vi "MGCC_FntStaMach_FlagCalculate_PhaseTwo.vi"(10 "Current SubMG":i32[](array[numeric]), 11 "Input State":string[](array[string])) -> (3 "Output Event":bool[][](array[boolean]))   [LabVIEW 2016]
uses:
  MGCC_FntStaMach_gobal.vi
  <vilib>/imath/engines/lvmath2/RunTimeEngine/IndexRead/NIMS M(S,$).vi
  <instcachedir>/0/NIMS M(S,$)_F24F360562DE41D8BE234322A2E15C65.lvgen/NIMS M(S,$)_F24F360562DE41D8BE234322A2E15C65_000.vi
  <vilib>/imath/engines/lvmath2/RunTimeEngine/BuiltInFunctions/length/NIMS_length(GV).vi
  <instcachedir>/0/NIMS_length(GV)_08A3D13377FD4E4B96F5795FBF3698FA.lvgen/NIMS_length(GV)_08A3D13377FD4E4B96F5795FBF3698FA_000.vi
  <vilib>/imathl/engines/lvmath/Functions/Error Handling/Create Error.vi
  <vilib>/imath/engines/lvmath2/RunTimeEngine/RangeToken/NIMS_Range_R3 - Integer.vi
  <instcachedir>/0/NIMS_Range_R3 - Integer_A435E2FF893B4C718FD5055FE39FE2F6.lvgen/NIMS_Range_R3 - Integer_A435E2FF893B4C718FD5055FE39FE2F6_000.vi
  <vilib>/imath/engines/lvmath2/RunTimeEngine/CommandStatement/MC_CommandStatement_break.vi
  <vilib>/imath/engines/lvmath2/RunTimeEngine/IndexRead/NIMS M(S,S).vi
  <instcachedir>/0/NIMS M(S,S)_AC51E74150A542F7991B9634C66F3096.lvgen/NIMS M(S,S)_AC51E74150A542F7991B9634C66F3096_000.vi
  <vilib>/imath/engines/lvmath2/RunTimeEngine/BuiltInFunctions/findnz/NIMS_[1o]_findnz(GRowV).vi
  <instcachedir>/0/NIMS_[1o]_findnz(GRowV)_1AF74843B4874134ADE908C0A4A72F3C.lvgen/NIMS_[1o]_findnz(GRowV)_1AF74843B4874134ADE908C0A4A72F3C_000.vi
  <vilib>/imath/engines/lvmath2/RunTimeEngine/BuiltInFunctions/is_empty/NIMS_is_empty(GV).vi
  <instcachedir>/0/NIMS_is_empty(GV)_FC7E7C3D9544432CB6AA2416ADCF6D56.lvgen/NIMS_is_empty(GV)_FC7E7C3D9544432CB6AA2416ADCF6D56_000.vi
  <vilib>/imath/engines/lvmath2/RunTimeEngine/ErrorHandling/NIMS_Create Error From Enums.vi
  <vilib>/imath/engines/lvmath2/RunTimeEngine/NodeEndStatement/NIMS_NodeEndStatement_Output.vi
  <instcachedir>/0/NIMS_NodeEndStatement_Output_53EC0D466D134D7ABD903AC30B43404B.lvgen/NIMS_NodeEndStatement_Output_53EC0D466D134D7ABD903AC30B43404B_013.vi
  <vilib>/imath/engines/lvmath2/RunTimeEngine/ErrorHandling/NIMS_Finalize Error.vi
panel:
  in  "ISD":bool
  out "Current SubMG":dbl
  out "Error Array":errorcluster[](array[cluster])
  in  "Ready for the next MG":bool
  in  "FLT 10":bool
  in  "ABN 10":bool
  in  "STD 6":bool
  in  "FLT 9":bool
  in  "ABN 9":bool
  in  "STD 5":bool
  in  "OFF":bool
  in  "GC 4":bool
  in  "ISD 6":bool
  in  "G2I_UN 3":bool
  in  "G2I_IN 3":bool
  in  "STD 4":bool
  in  "I2G 3":bool
  in  "BKS 3":bool
  in  "ABN 8":bool
  in  "FLT 8":bool
  in  "STD 3":bool
  in  "BKS 2":bool
  in  "ABN 7":bool
  in  "FLT 7":bool
  in  "ISD 5":bool
  in  "STD  3":bool
  in  "I2G 2":bool
  in  "ABN 6":bool
  in  "FLT 6":bool
  in  "GC 3":bool
  in  "STD 2":bool
  in  "ISD 4":bool
  in  "ABN 5":bool
  in  "FLT 5":bool
  in  "G2I_UN 2":bool
  in  "STD  2":bool
  in  "ISD 3":bool
  in  "ABN 4":bool
  in  "FLT 4":bool
  in  "G2I_IN 2":bool
  in  "I2G":bool
  in  "ISD 2":bool
  in  "ABN 3":bool
  in  "FLT 3":bool
  in  "GC 2":bool
  in  "G2I_UN":bool
  in  "G2I_IN":bool
  in  "ABN 2":bool
  in  "FLT 2":bool
  in  "GC":bool
  in  "ISD":bool
  in  "BKS":bool
  in  "STD":bool
  in  "ABN":bool
  in  "FLT":bool
  # "OFF State"
  # "STD State"
  # "GC State"
  # "BKS State"
  # "ISD State"
  # "ABN State"
  # "G2I_UN State"
  # "G2I_IN State"
  # "FLT State"
  # "I2G State"
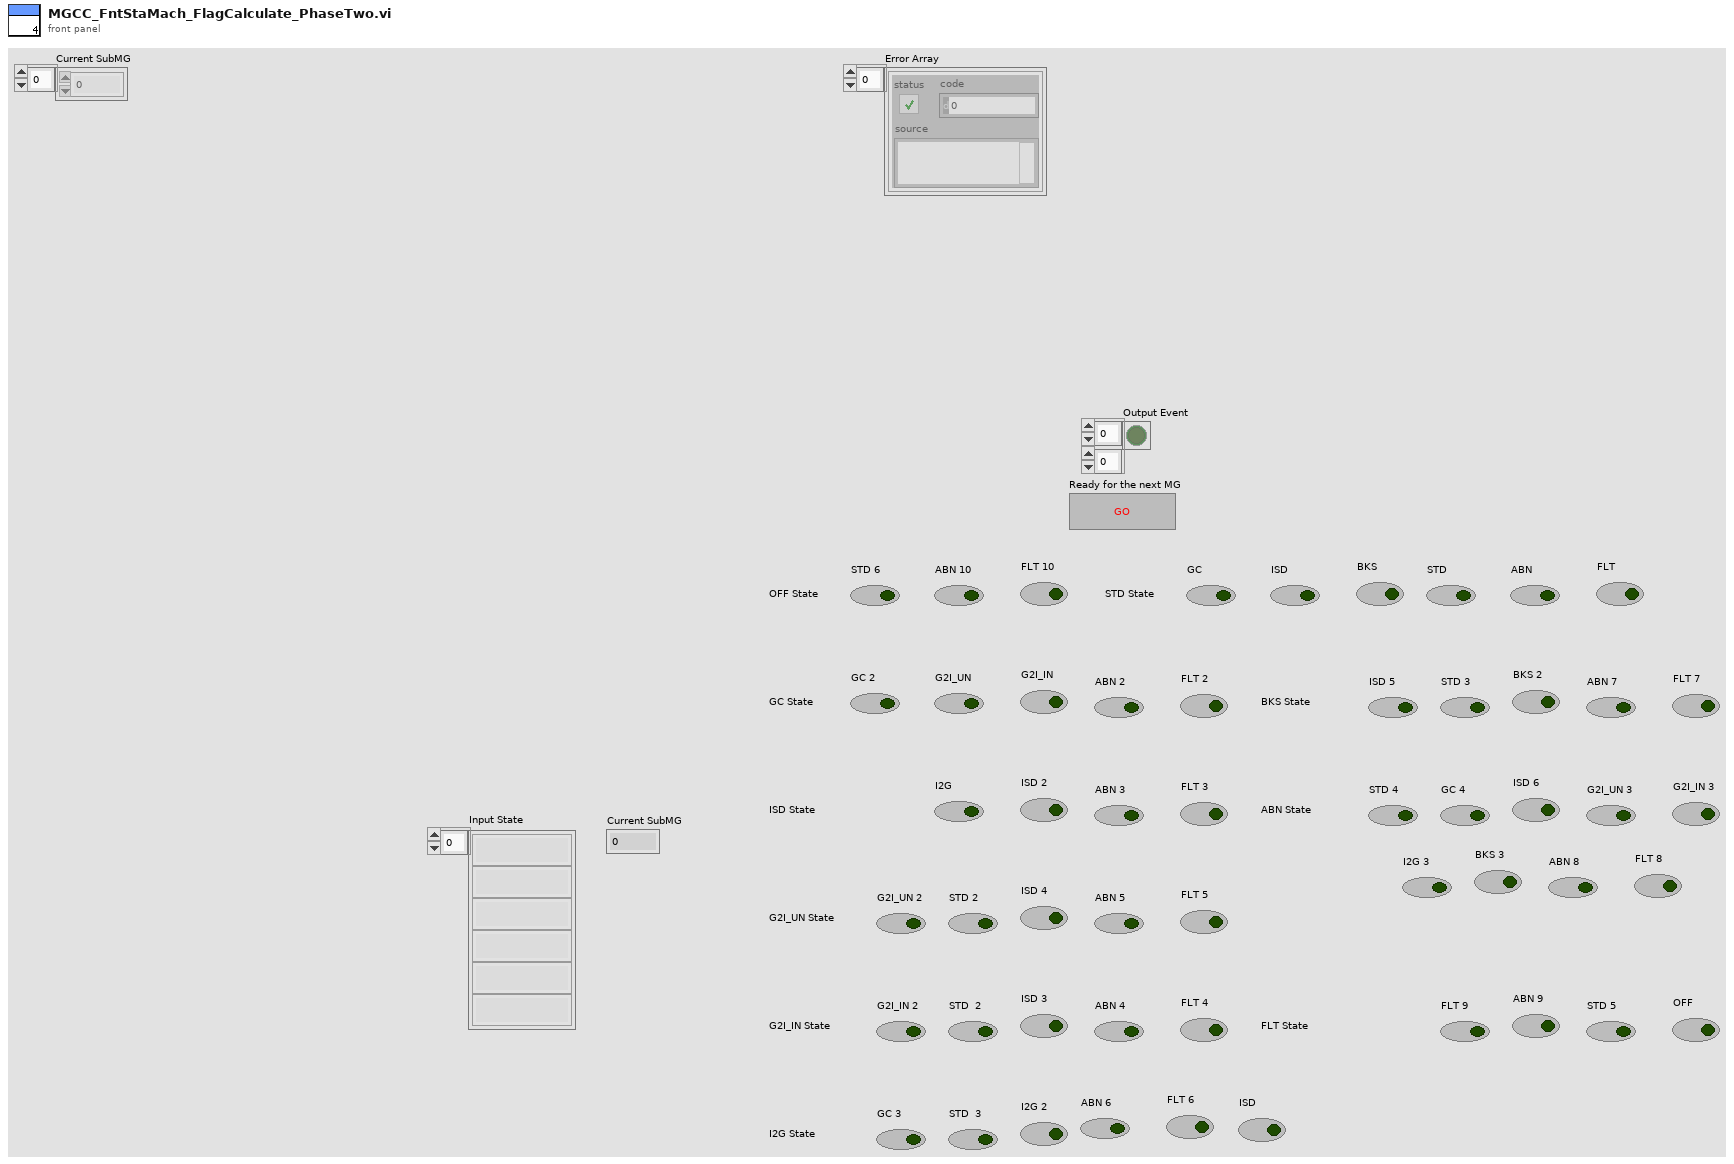
[diagram p1: front panel]
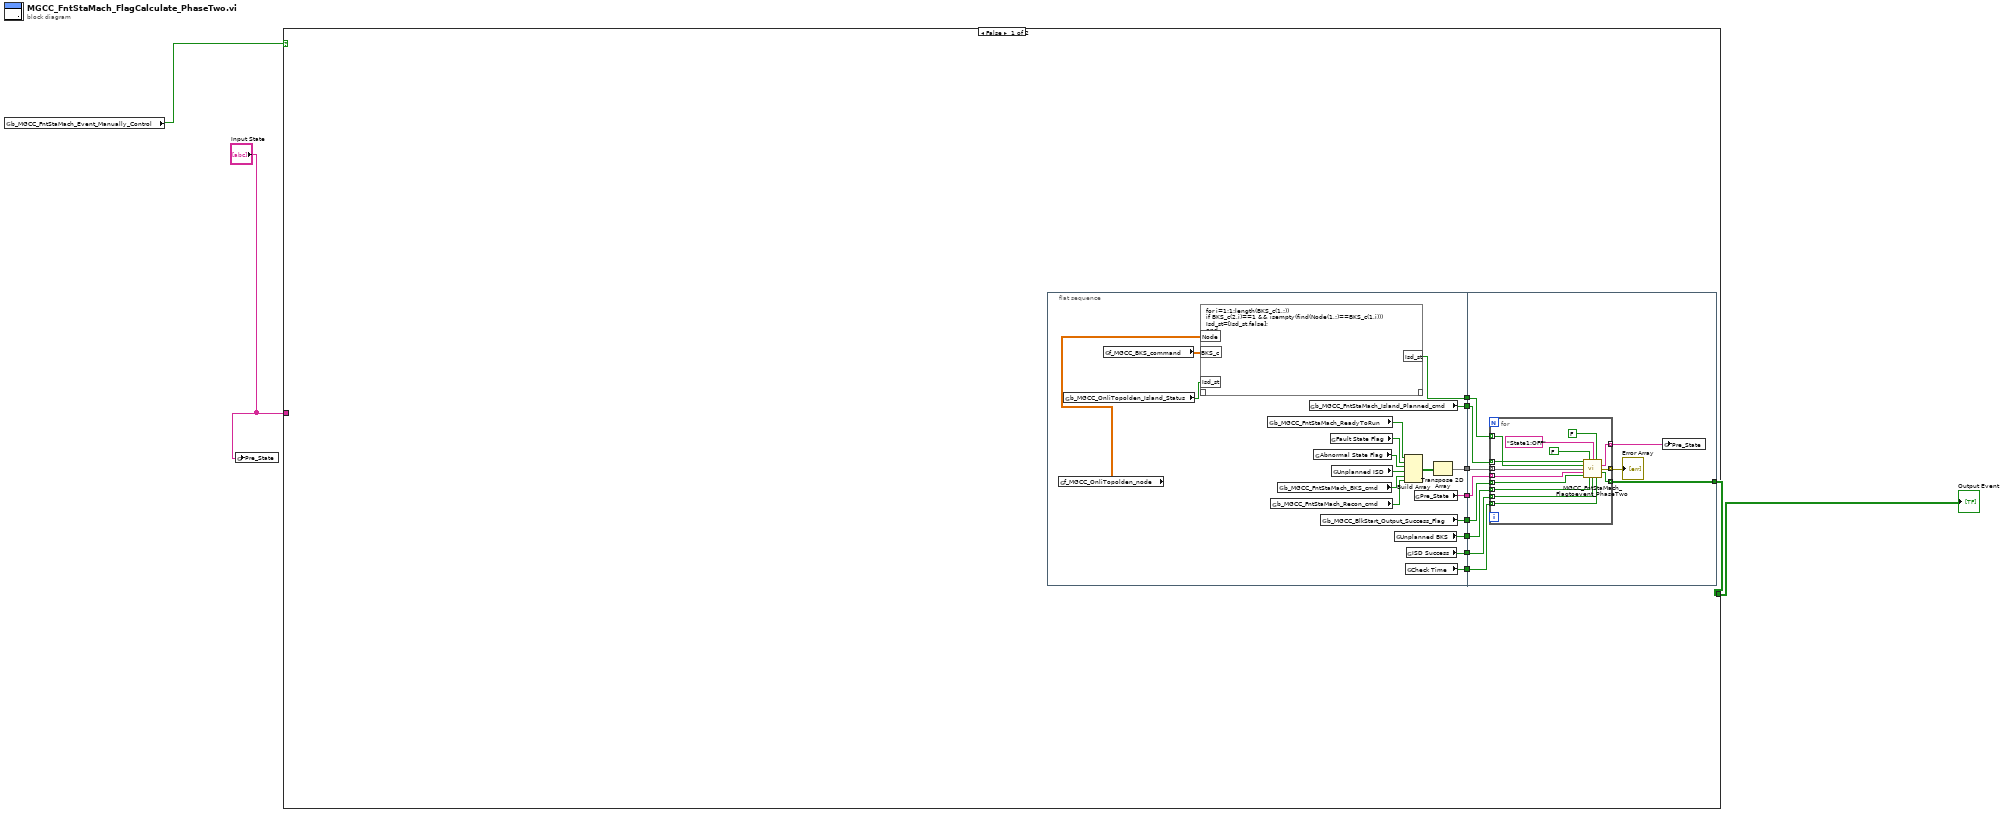
[diagram p0: block diagram]
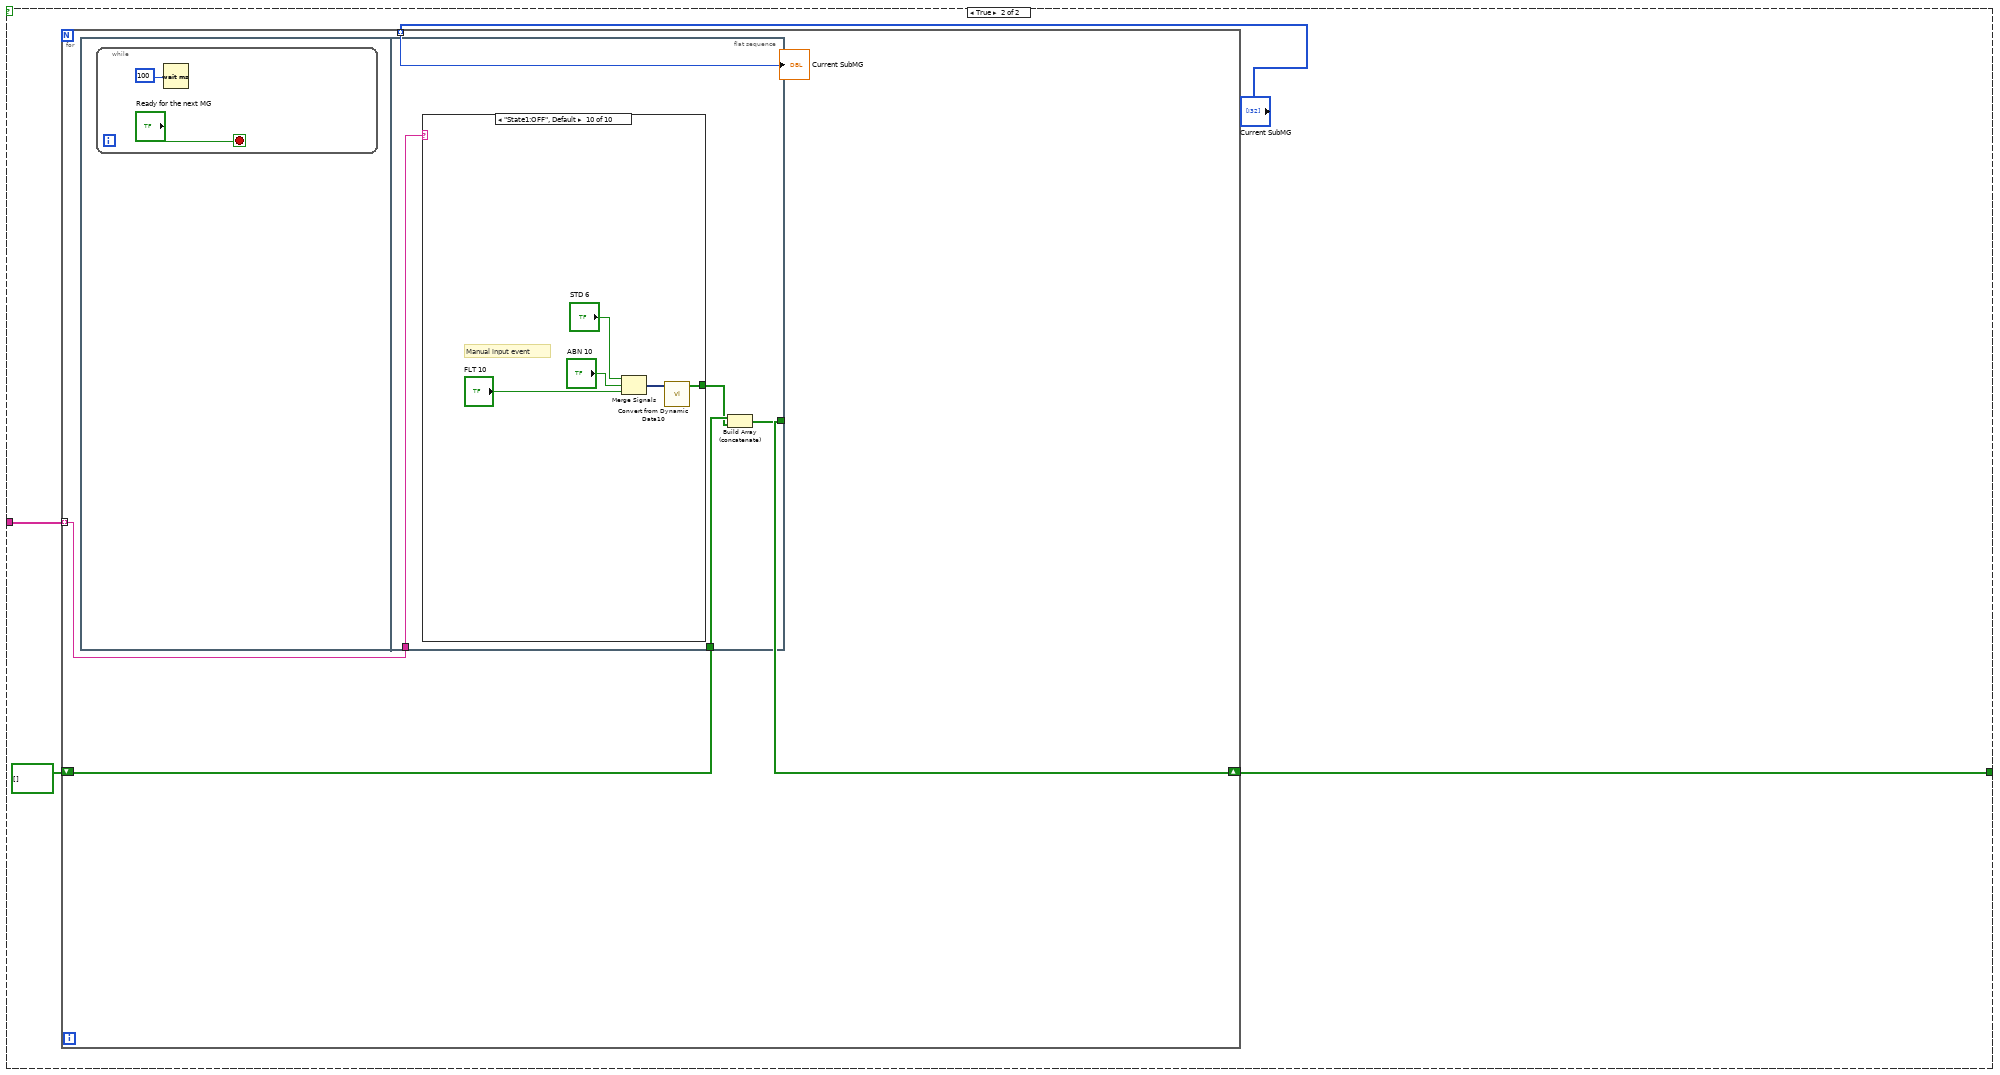
[diagram p2: hidden frame]
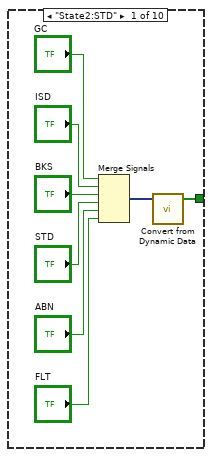
[diagram p3: hidden frame]
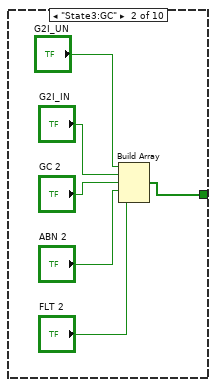
[diagram p4: hidden frame]
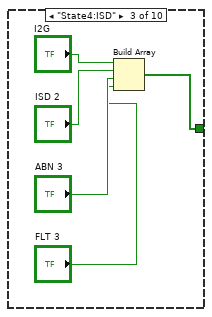
[diagram p5: hidden frame]
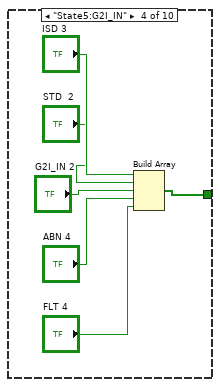
[diagram p6: hidden frame]
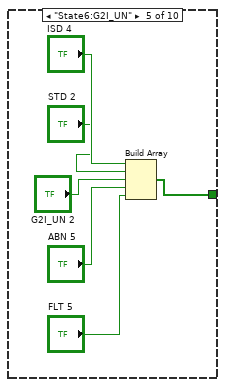
[diagram p7: hidden frame]
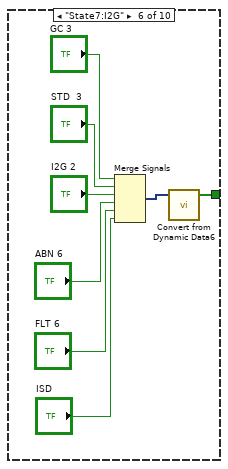
[diagram p8: hidden frame]
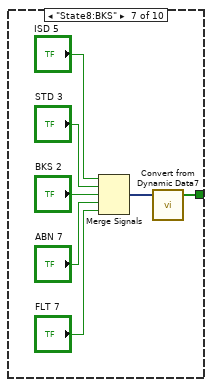
[diagram p9: hidden frame]
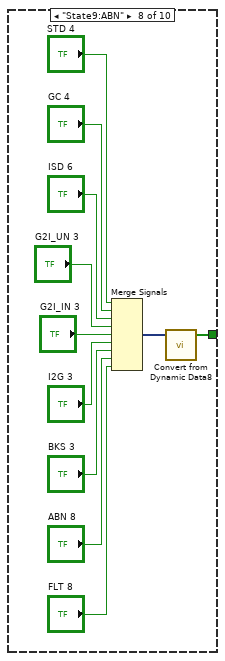
[diagram p10: hidden frame]
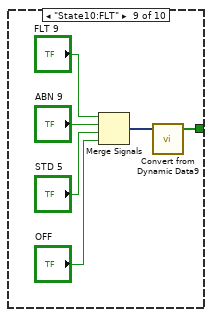
[diagram p11: hidden frame]
diagram:
  n1 = global read "MGCC_FntStaMach_gobal.vi" "b_MGCC_FntStaMach_Event_Manually_Control"() -> (w3:bool)
  n2 = global write "MGCC_FntStaMach_gobal.vi" "Pre_State"("Input State") -> ()
  n3 = case shown="False" w3 {
    tunnel: "Input State" -> [_ w197]
    tunnel: [w4 w194] -> w2
    frame False {
      n4 = flat-sequence {
        tunnel: [w17] -> w12
        tunnel: [w24] -> w11
        tunnel: [w14] -> w10
        tunnel: [w23] -> w9
        tunnel: [w22] -> w8
        tunnel: [w21] -> w7
        tunnel: [w20] -> w6
        tunnel: [w19] -> w5
        tunnel: w12 -> [w179]
        tunnel: w11 -> [w178]
        tunnel: w10 -> [w177]
        tunnel: w9 -> [w176]
        tunnel: w8 -> [w175]
        tunnel: w7 -> [w174]
        tunnel: w6 -> [w173]
        tunnel: w5 -> [w172]
        tunnel: [w170] -> w4
        frame #0 {
          n5 = global read "MGCC_FntStaMach_gobal.vi" "f_MGCC_OnliTopolden_node"() -> (w13:dbl[][])
          n6 = global read "MGCC_FntStaMach_gobal.vi" "b_MGCC_OnliTopolden_Island_Status"() -> (w15:bool[])
          n7 = global read "MGCC_FntStaMach_gobal.vi" "f_MGCC_BKS_command"() -> (w16:dbl[][])
          n8 = mathscript code="for i=1:1:length(BKS_c(1,:))\nif BKS_c(2,i)==1 && isempty(find(Node(1,:)==BKS_c(1,i)))\nIsd_st=[Isd_st,false];\nend\nend"("BKS_c"=w16, "Isd_st"=w15, "Node"=w13) -> ("Isd_st"=w14:bool[])  [unwired: 1 in, 1 out]
          n9 = global read "MGCC_FntStaMach_gobal.vi" "b_MGCC_FntStaMach_ReadyToRun"() -> (w30:bool[])
          n10 = global read "MGCC_FntStaMach_gobal.vi" "b_MGCC_FntStaMach_Recon_cmd"() -> (w25:bool[])
          n11 = global read "MGCC_FntStaMach_gobal.vi" "b_MGCC_FntStaMach_BKS_cmd"() -> (w26:bool[])
          n12 = global read "MGCC_FntStaMach_gobal.vi" "b_MGCC_FntStaMach_Island_Planned_cmd"() -> (w24:bool[])
          n13 = global read "MGCC_FntStaMach_gobal.vi" "Abnormal State Flag"() -> (w28:bool[])
          n14 = global read "MGCC_FntStaMach_gobal.vi" "b_MGCC_BlkStart_Output_Success_Flag"() -> (w22:bool[])
          n15 = global read "MGCC_FntStaMach_gobal.vi" "Fault State Flag"() -> (w29:bool[])
          n16 = global read "MGCC_FntStaMach_gobal.vi" "Unplanned ISD"() -> (w27:bool[])
          n17 = global read "MGCC_FntStaMach_gobal.vi" "Unplanned BKS"() -> (w21:bool[])
          n18 = Build Array(w30, w29, w28, w27, w26, w25) -> (w18:bool[][])
          n19 = global read "MGCC_FntStaMach_gobal.vi" "Check Time"() -> (w19:bool[])
          n20 = global read "MGCC_FntStaMach_gobal.vi" "ISD Success"() -> (w20:bool[])
          n21 = global read "MGCC_FntStaMach_gobal.vi" "Pre_State"() -> (w23:string[])
          n22 = Transpose 2D Array(2D array=w18) -> (transposed array=w17:bool[][])
        }
        frame #1 {
          n23 = for {
            tunnel: w179 -> [w193] mode=indexing
            tunnel: w178 -> [w192] mode=indexing
            tunnel: w177 -> [w191] mode=indexing
            tunnel: w176 -> [w190] mode=indexing
            tunnel: w175 -> [w189] mode=indexing
            tunnel: w174 -> [w185] mode=indexing
            tunnel: w173 -> [w184] mode=indexing
            tunnel: w172 -> [w183] mode=indexing
            tunnel: [w182] -> w171 mode=indexing
            tunnel: [w181] -> w170 mode=indexing
            tunnel: [w180] -> w169 mode=indexing
            n24 = call "MGCC_FntStaMach_Flagtoevent_PhaseTwo.vi"("Island_status"=w191, "M_OFF"=FALSE, "ABN_state"="State1:OFF", "ABN_recover"=FALSE, "planned_isd"=w192, "Flags"=w193, "Pre_state"=w190, "BKS_s"=w189, "UnplanBKS"=w185, "ISD_success"=w184, "Check_time"=w183) -> ("Previous_state"=w180:string, "error out"=w182:errorcluster, "Event"=w181:bool[])  [unwired: 2 in]
          }
          "Error Array" <- w171
          n25 = global write "MGCC_FntStaMach_gobal.vi" "Pre_State"(w169) -> ()
        }
      }
    }
    frame True {
      n26 = for {
        tunnel: w197 -> [w200] mode=indexing
        tunnel: "Current SubMG" -> [w201] mode=indexing
        shift-right: [w198] -> w194
        shift-left: bool[][] [] -> [w199]
        n27 = flat-sequence {
          tunnel: w200 -> [w207]
          tunnel: w199 -> [w205]
          tunnel: [w206] -> w198
          frame #0 {
            n28 = while {
              stop <- "Ready for the next MG" stop-if-true
              n29 = Wait (ms)(milliseconds to wait=u32 100) -> ()  [unwired: 1 out]
            }
          }
          frame #1 {
            n30 = case shown="\"State1:OFF\", Default" w207 {
              tunnel: [w208 w216 w222 w227 w233 w240 w247 w254 w265 w271] -> w204
              frame "State2:STD" {
                n31 = Merge Signals("GC", "ISD", "BKS", "STD", "ABN", "FLT") -> (w209:dynamicdata)
                n32 = call "Convert from Dynamic Data"("Dynamic Data Type"=w209) -> ("Array"=w208:bool[])  [unwired: 3 in]
              }
              frame "State3:GC" {
                n33 = Build Array("G2I_UN", "G2I_IN", "GC 2", "ABN 2", "FLT 2") -> (w216:bool[])
              }
              frame "State4:ISD" {
                n34 = Build Array("I2G", "ISD 2", "ABN 3", "FLT 3") -> (w222:bool[])
              }
              frame "State5:G2I_IN" {
                n35 = Build Array("ISD 3", "STD  2", "G2I_IN 2", "ABN 4", "FLT 4") -> (w227:bool[])
              }
              frame "State6:G2I_UN" {
                n36 = Build Array("ISD 4", "STD 2", "G2I_UN 2", "ABN 5", "FLT 5") -> (w233:bool[])
              }
              frame "State7:I2G" {
                n37 = Merge Signals("GC 3", "STD  3", "I2G 2", "ABN 6", "FLT 6", "ISD") -> (w241:dynamicdata)
                n38 = call "Convert from Dynamic Data6"("Dynamic Data Type"=w241) -> ("Array"=w240:bool[])  [unwired: 3 in]
              }
              frame "State8:BKS" {
                n39 = Merge Signals("ISD 5", "STD 3", "BKS 2", "ABN 7", "FLT 7") -> (w248:dynamicdata)
                n40 = call "Convert from Dynamic Data7"("Dynamic Data Type"=w248) -> ("Array"=w247:bool[])  [unwired: 3 in]
              }
              frame "State9:ABN" {
                n41 = Merge Signals("STD 4", "GC 4", "ISD 6", "G2I_UN 3", "G2I_IN 3", "I2G 3", "BKS 3", "ABN 8", "FLT 8") -> (w255:dynamicdata)
                n42 = call "Convert from Dynamic Data8"("Dynamic Data Type"=w255) -> ("Array"=w254:bool[])  [unwired: 3 in]
              }
              frame "State10:FLT" {
                n43 = Merge Signals("FLT 9", "ABN 9", "STD 5", "OFF") -> (w266:dynamicdata)
                n44 = call "Convert from Dynamic Data9"("Dynamic Data Type"=w266) -> ("Array"=w265:bool[])  [unwired: 3 in]
              }
              frame "State1:OFF", Default {
                # "Manual input event"
                n45 = Merge Signals("STD 6", "ABN 10", "FLT 10") -> (w272:dynamicdata)
                n46 = call "Convert from Dynamic Data10"("Dynamic Data Type"=w272) -> ("Array"=w271:bool[])  [unwired: 3 in]
              }
            }
            n47 = Build Array (concatenate)(w205, w204) -> (w206:bool[][])
          }
        }
        "Current SubMG" <- w201
      }
    }
  }
  "Output Event" <- w2
